vi "dfd_Generate Target Filter Path.vi"(8 "error in (no error)":errorcluster, 10 "destination path":path, 11 "filter name":string) -> (0 "error out":errorcluster, 1 "project folder name":string, 2 "target VI path":path, 3 "dup filter name":string)   [LabVIEW 2017, in "NI_DigFilterLicensed.lvlib"]
uses:
  <vilib>/addons/Digital Filter Design/NI_DigFilterLicensed.lvlib
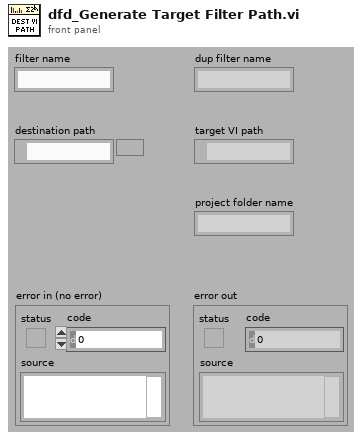
[diagram p1: front panel]
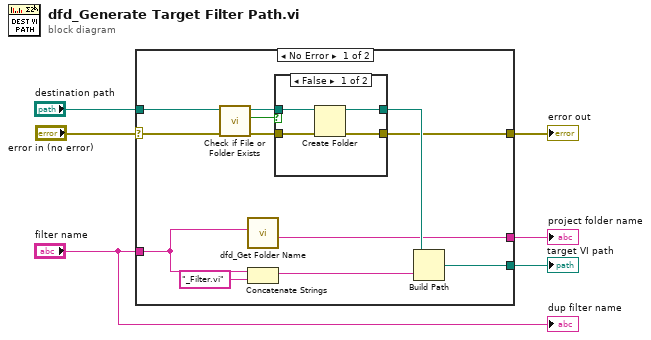
[diagram p0: block diagram]
diagram:
  n1 = case shown="No Error" "error in (no error)" {
    selector: "error in (no error)" -> [w10 w25]
    tunnel: [w18 _] -> w6
    tunnel: [w7 _] -> w5
    tunnel: "destination path" -> [w9 _]
    tunnel: "filter name" -> [w8 _]
    tunnel: [w11 w25] -> w2
    frame No Error {
      n2 = call <vilib>:"Check if File or Folder Exists.vi"("error in (no error)"=w10, "path"=w9) -> ("error out"=w13:errorcluster, "file or folder exists?"=w15:bool, "dup path"=w14:path)  [unwired: 7 out]
      n3 = call <vilib>:"dfd_Get Folder Name.vi"("filter name"=w8) -> ("folder name"=w7:string)  [unwired: 10 out]
      n4 = Concatenate Strings(w8, "_Filter.vi" ("string")) -> (w17:string)
      n5 = case shown="False" w15 {
        tunnel: w14 -> [w22 w24]
        tunnel: [w19 w24] -> w12
        tunnel: w13 -> [w21 w23]
        tunnel: [w20 w23] -> w11
        frame False {
          n6 = Create Folder(path (use dialog)=w22, error in=w21) -> (created path=w19:path, error out=w20:errorcluster)  [unwired: 2 out]
        }
        frame True {
        }
      }
      n7 = Build Path(base path=w12, name or relative path=w17) -> (appended path=w18:path)
    }
    frame Error {
    }
  }
  "target VI path" <- w6
  "project folder name" <- w5
  "error out" <- w2
  "dup filter name" <- "filter name"
